vi "LV to text.vi"() -> ()   [LabVIEW 2013]
uses:
  <vilib>/_script/All Supported PropertiesOrMethods TypeDefs/ASC_ArrayOfUniqueIDStringParentIDStringName.ctl
  <vilib>/_script/All Supported PropertiesOrMethods TypeDefs/ASC_UniqueIDStringParentIDStringName.ctl
panel:
  out "Array 5":cluster{i32, "AllTypes[]":T1, "Type":T2}[](array[cluster])
  out "Array 4":cluster{i32, refnum<vi>}[](array[cluster])
  out "const":T3(array[cluster])
  out "Array 2":bool[][](array[boolean])
  out "Array":T4(array[cluster])
  out "nodes":T5(array[cluster])
  out "connectorPane":T6(array[cluster])
  out "NConn":u32
  out "Pattern":u32
  out "SubVIs":T7(array[cluster])
  out "AllObj":T8(array[cluster])
  out "Decorations[]":refnum<vi>[](array[refnum])
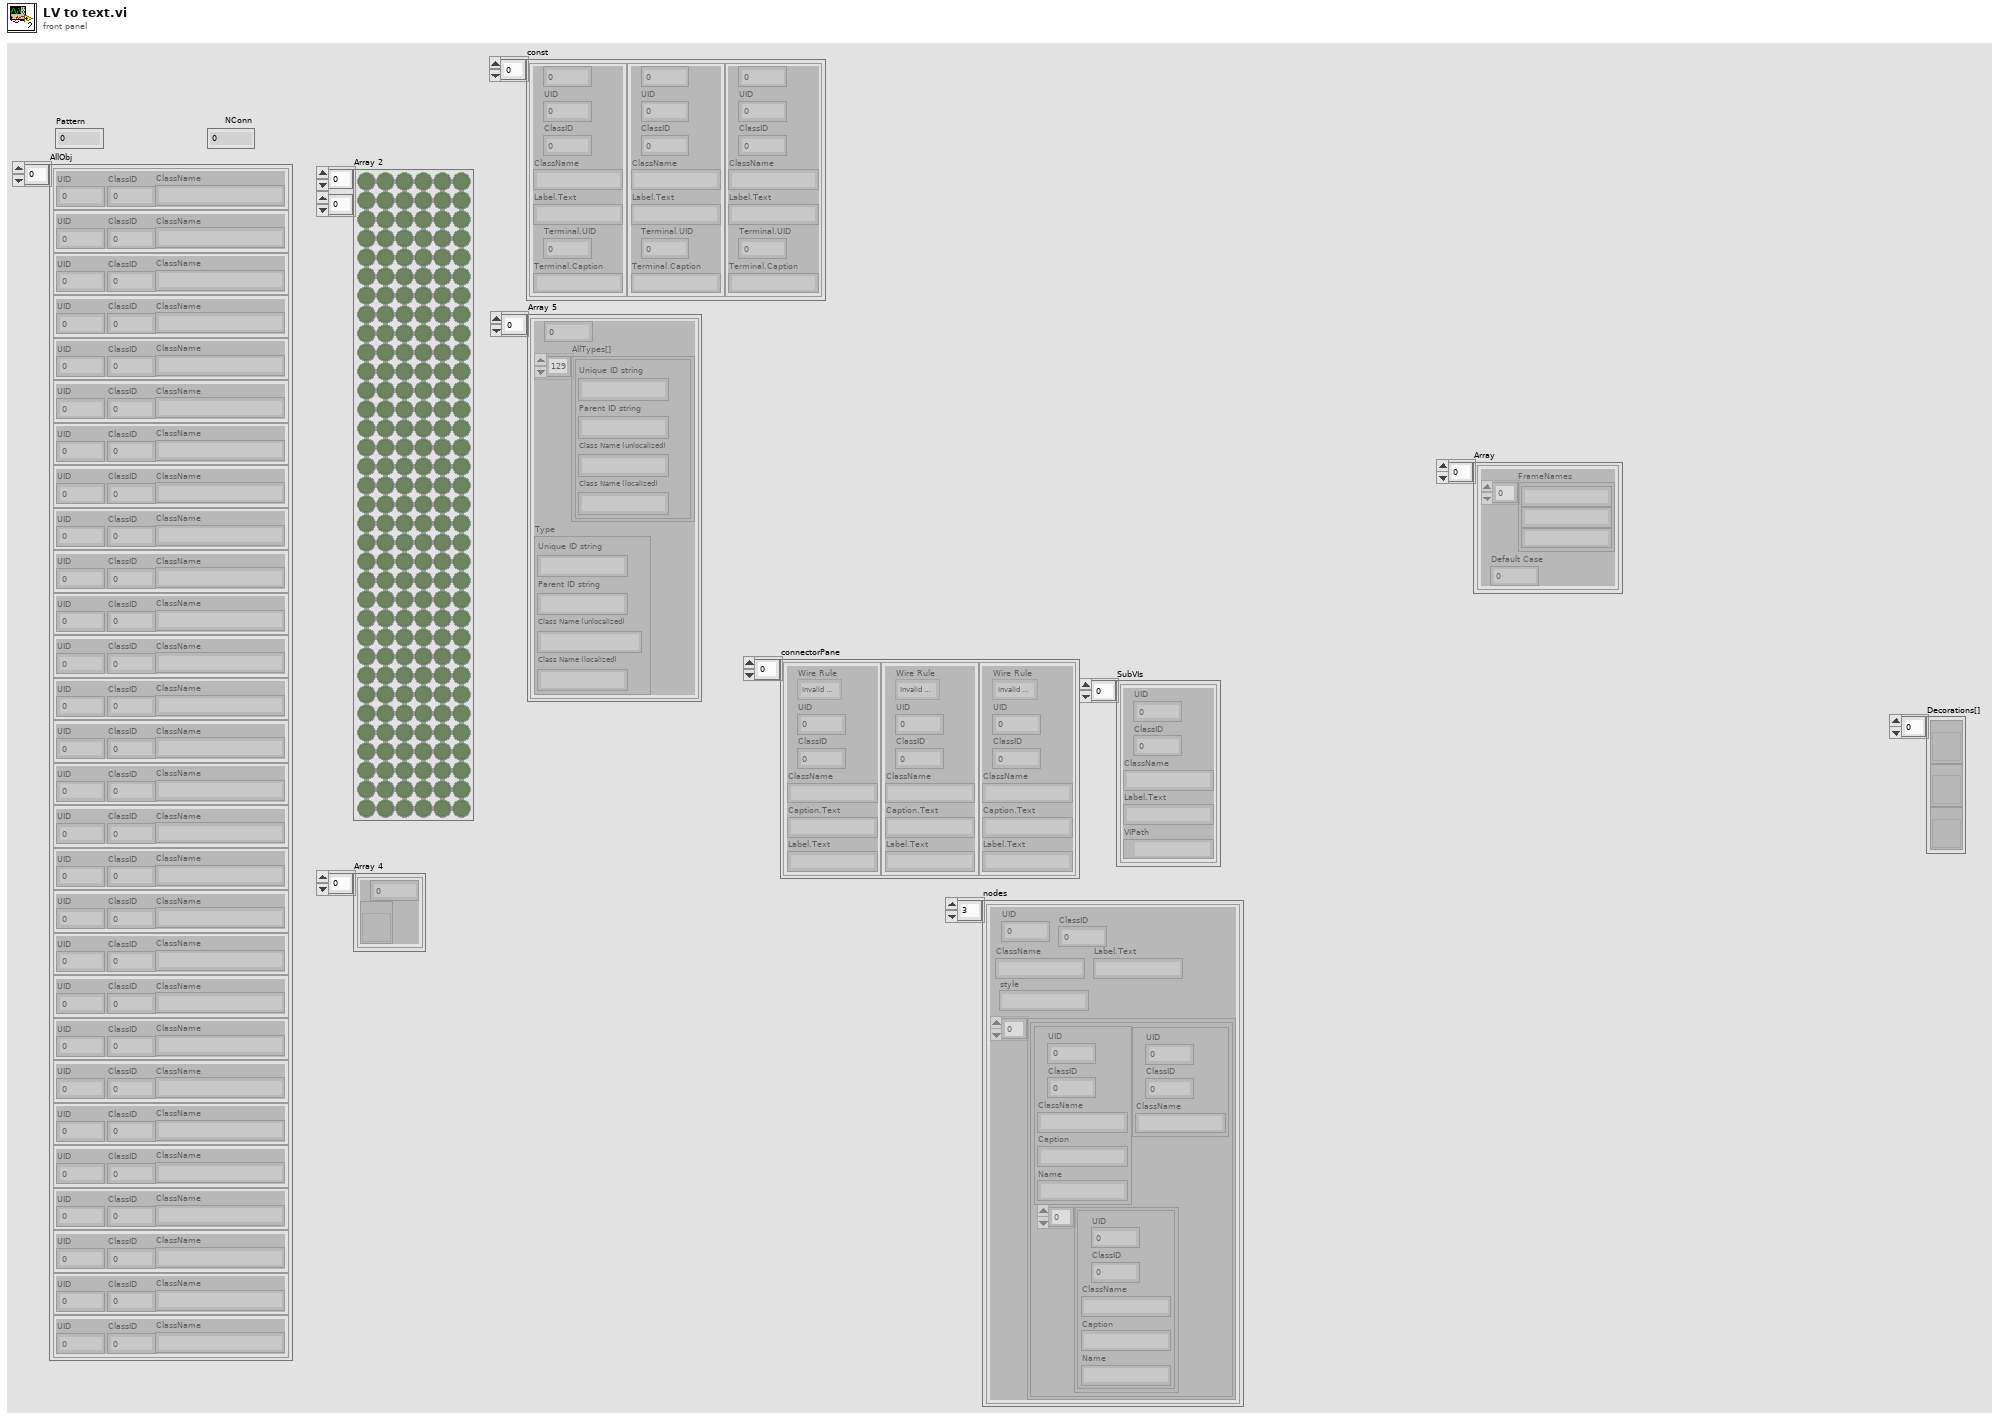
[diagram p1: front panel]
types:
  T1 = typedef "ASC_ArrayOfUniqueIDStringParentIDStringName.ctl" = T2[]
  T2 = typedef "ASC_UniqueIDStringParentIDStringName.ctl" = cluster{"Unique ID string":string, "Parent ID string":string, "Class Name (unlocalized)":string, "Class Name (localized)":string}
  T3 = cluster{i32, "UID":i32, "ClassID":u32, "ClassName":string, "Label.Text":string, "Terminal.UID":i32, "Terminal.Caption":string}[]
  T4 = cluster{"FrameNames":string[], "Default Case":i32}[]
  T5 = cluster{"UID":i32, "ClassID":u32, "ClassName":string, "Label.Text":string, "style":string, cluster{cluster{"UID":i32, "ClassID":u32, "ClassName":string, "Caption":string, "Name":string}, cluster{"UID":i32, "ClassID":u32, "ClassName":string}, cluster{"UID":i32, "ClassID":u32, "ClassName":string, "Caption":string, "Name":string}[]}[]}[]
  T6 = cluster{"Wire Rule":enum16{"Invalid Wire Rule", "Required", "Recommended", "Optional", "Dynamic Dispatch"}, "UID":i32, "ClassID":u32, "ClassName":string, "Caption.Text":string, "Label.Text":string}[]
  T7 = cluster{"UID":i32, "ClassID":u32, "ClassName":string, "Label.Text":string, "VIPath":path}[]
  T8 = cluster{"UID":i32, "ClassID":u32, "ClassName":string}[]
  T9 = enum16{"Invalid Wire Rule", "Required", "Recommended", "Optional", "Dynamic Dispatch"}[]
  T10 = cluster{"Wire Rule":enum16{"Invalid Wire Rule", "Required", "Recommended", "Optional", "Dynamic Dispatch"}, "UID":i32, "ClassID":u32, "ClassName":string, "Caption.Text":string, "Label.Text":string}
  T11 = cluster{"UID":i32, "ClassID":u32, "ClassName":string}
  T12 = cluster{"UID":i32, "ClassID":u32, "ClassName":string, "Caption":string, "Name":string}
  T13 = cluster{cluster{"UID":i32, "ClassID":u32, "ClassName":string, "Caption":string, "Name":string}, cluster{"UID":i32, "ClassID":u32, "ClassName":string}, cluster{"UID":i32, "ClassID":u32, "ClassName":string, "Caption":string, "Name":string}[]}
  T14 = cluster{"UID":i32, "ClassID":u32, "ClassName":string, "Label.Text":string, "Style":string, cluster{cluster{"UID":i32, "ClassID":u32, "ClassName":string, "Caption":string, "Name":string}, cluster{"UID":i32, "ClassID":u32, "ClassName":string}, cluster{"UID":i32, "ClassID":u32, "ClassName":string, "Caption":string, "Name":string}[]}[]}
  T15 = cluster{"UID":i32, "ClassID":u32, "ClassName":string, "Label.Text":string, "VIPath":path}
  T16 = cluster{i32, "UID":i32, "ClassID":u32, "ClassName":string, "Label.Text":string, "Terminal.UID":i32, "Terminal.Caption":string}
  T17 = cluster{"FrameNames":string[], "Default Case":i32}
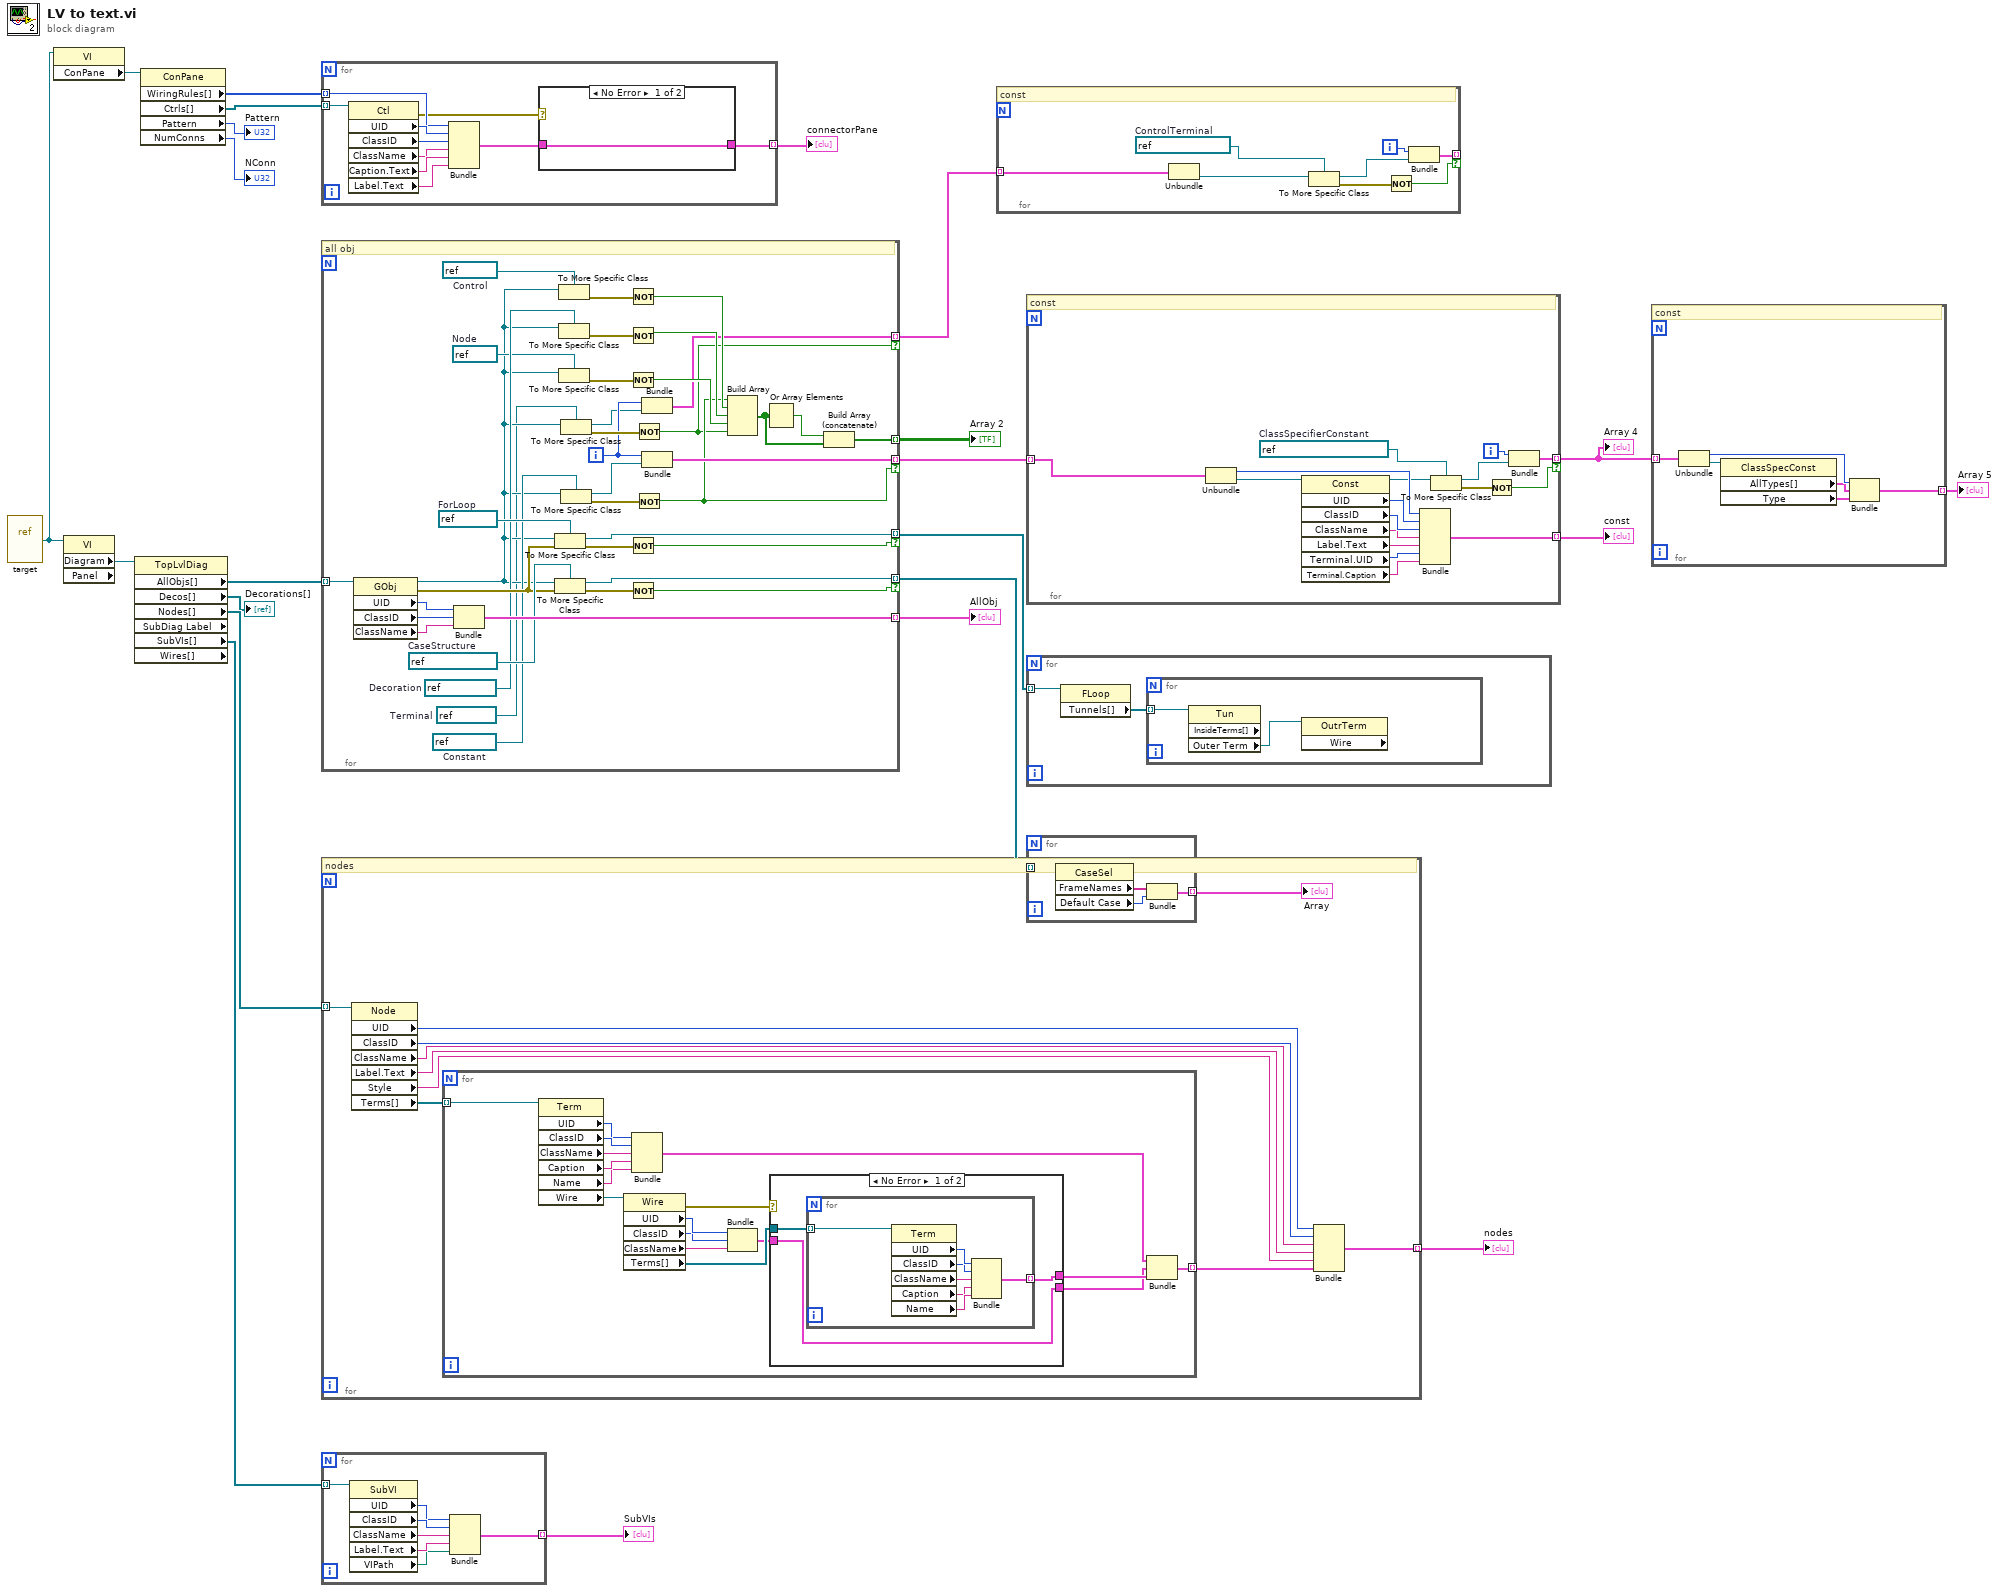
[diagram p0: block diagram]
diagram:
  n1 = vi-ref "target.vi"() -> (w24:refnum<vi>)
  n2 = property class="VI"(reference=w24) -> ("ConPane"=w17:refnum<vi>)  [unwired: 1 in, 2 out]
  n3 = property class="VI" props=["Diagram", "Panel"](reference=w24) -> ("Diagram"=w23:refnum<vi>)  [unwired: 1 in, 3 out]
  n4 = property class="TopLvlDiag" props=["AllObjs[]", "Decos[]", "Nodes[]", "SubDiag Label", "SubVIs[]", "Wires[]"](reference=w23) -> ("AllObjs[]"=w7:refnum<vi>[], "Decos[]"=→"Decorations[]":refnum<vi>[], "Nodes[]"=w22:refnum<vi>[], "SubVIs[]"=w20:refnum<vi>[])  [unwired: 1 in, 4 out]
  n5 = property class="ConPane"(reference=w17) -> ("WiringRules[]"=w14:T9, "Ctrls[]"=w13:refnum<vi>[], "Pattern"=→"Pattern":u32, "NumConns"=→"NConn":u32)  [unwired: 1 in, 2 out]
  n6 = for {
    tunnel: w14 -> [w28] mode=indexing
    tunnel: w13 -> [w29] mode=indexing
    tunnel: [w25] -> w12 mode=indexing
    n7 = property class="Ctl"(reference=w29) -> (error out=w27:errorcluster, "UID"=w30:i32, "ClassID"=w31:u32, "ClassName"=w32:string, "Caption.Text"=w33:string, "Label.Text"=w34:string)  [unwired: 1 in, 1 out]
    n8 = Bundle("Wire Rule"=w28, "UID"=w30, "ClassID"=w31, "ClassName"=w32, "Caption.Text"=w33, "Label.Text"=w34) -> (w26:T10)  [unwired: 1 in]
    n9 = case shown="No Error" w27 {
      tunnel: w26 -> [w35 _]
      tunnel: [w35 _] -> w25
      frame No Error {
      }
      frame Error {
      }
    }
  }
  "connectorPane" <- w12
  n10 = for {
    tunnel: w7 -> [w62] mode=indexing
    tunnel: [w71] -> w19 mode=indexing
    tunnel: [w68] -> w10 mode=indexing if=w52
    tunnel: [w64] -> w8 mode=indexing if=w53
    tunnel: [w41] -> w6 mode=indexing
    tunnel: [w44] -> w5 mode=indexing if=w38
    tunnel: [w39] -> w1 mode=indexing if=w36
    i -> [w40]
    w47 = refnum<vi> refnum  # Terminal
    w58 = refnum<vi> refnum  # Node
    w59 = refnum<vi> refnum  # Decoration
    w60 = refnum<vi> refnum  # Control
    w61 = refnum<vi> refnum  # Constant
    w66 = refnum<vi> refnum  # ForLoop
    w69 = refnum<vi> refnum  # CaseStructure
    # "all obj"
    n11 = property class="GObj"(reference=w62) -> (reference out=w48:refnum<vi>, error out=w65:errorcluster, "UID"=w70:i32, "ClassID"=w73:u32, "ClassName"=w72:string)  [unwired: 1 in]
    n12 = Bundle("UID"=w70, "ClassID"=w73, "ClassName"=w72) -> (w71:T11)  [unwired: 1 in]
    n13 = To More Specific Class(target class=w66, reference=w48, error in=w65) -> (specific class reference=w64:refnum<vi>, error out=w63:errorcluster)
    n14 = To More Specific Class(target class=w69, reference=w48, error in=w65) -> (specific class reference=w68:refnum<vi>, error out=w67:errorcluster)
    n15 = To More Specific Class(target class=w60, reference=w48) -> (error out=w56:errorcluster)  [unwired: 1 in, 1 out]
    n16 = To More Specific Class(target class=w59, reference=w48) -> (error out=w55:errorcluster)  [unwired: 1 in, 1 out]
    n17 = To More Specific Class(target class=w58, reference=w48) -> (error out=w54:errorcluster)  [unwired: 1 in, 1 out]
    n18 = To More Specific Class(target class=w47, reference=w48) -> (specific class reference=w37:refnum<vi>, error out=w46:errorcluster)  [unwired: 1 in]
    n19 = To More Specific Class(target class=w61, reference=w48) -> (specific class reference=w45:refnum<vi>, error out=w57:errorcluster)  [unwired: 1 in]
    n20 = Not(x=w56) -> (.not. x?=w51:bool)
    n21 = Not(x=w55) -> (.not. x?=w50:bool)
    n22 = Not(x=w54) -> (.not. x?=w49:bool)
    n23 = Not(x=w63) -> (.not. x?=w53:bool)
    n24 = Not(x=w67) -> (.not. x?=w52:bool)
    n25 = Not(x=w46) -> (.not. x?=w36:bool)
    n26 = Not(x=w57) -> (.not. x?=w38:bool)
    n27 = Bundle(w40, w37) -> (w39:cluster{i32, refnum<vi>})  [unwired: 1 in]
    n28 = Bundle(w40, w45) -> (w44:cluster{i32, refnum<vi>})  [unwired: 1 in]
    n29 = Build Array(w38, w51, w50, w49, w36) -> (w43:bool[])
    n30 = Or Array Elements(Boolean array=w43) -> (logical OR=w42:bool)
    n31 = Build Array (concatenate)(w42, w43) -> (w41:bool[])
  }
  "AllObj" <- w19
  "Array 2" <- w6
  n32 = for {
    tunnel: w22 -> [w77] mode=indexing
    tunnel: [w80] -> w11 mode=indexing
    # "nodes"
    n33 = property class="Node"(reference=w77) -> ("UID"=w76:i32, "ClassID"=w82:u32, "ClassName"=w81:string, "Label.Text"=w79:string, "Style"=w74:string, "Terms[]"=w78:refnum<vi>[])  [unwired: 1 in, 2 out]
    n34 = for {
      tunnel: w78 -> [w99] mode=indexing
      tunnel: [w87] -> w75 mode=indexing
      n35 = property class="Term"(reference=w99) -> ("UID"=w94:i32, "ClassID"=w98:u32, "ClassName"=w97:string, "Caption"=w96:string, "Name"=w95:string, "Wire"=w93:refnum<vi>)  [unwired: 1 in, 2 out]
      n36 = property class="Wire"(reference=w93) -> (error out=w83:errorcluster, "UID"=w92:i32, "ClassID"=w91:u32, "ClassName"=w90:string, "Terms[]"=w89:refnum<vi>[])  [unwired: 1 in, 1 out]
      n37 = Bundle("UID"=w94, "ClassID"=w98, "ClassName"=w97, "Caption"=w96, "Name"=w95) -> (w88:T12)  [unwired: 1 in]
      n38 = Bundle("UID"=w92, "ClassID"=w91, "ClassName"=w90) -> (w85:T11)  [unwired: 1 in]
      n39 = case shown="No Error" w83 {
        tunnel: w89 -> [w102 _]
        tunnel: [w101 _] -> w86
        tunnel: w85 -> [w100 _]
        tunnel: [w100 _] -> w84
        frame No Error {
          n40 = for {
            tunnel: w102 -> [w104] mode=indexing
            tunnel: [w103] -> w101 mode=indexing
            n41 = property class="Term"(reference=w104) -> ("UID"=w109:i32, "ClassID"=w105:u32, "ClassName"=w106:string, "Caption"=w107:string, "Name"=w108:string)  [unwired: 1 in, 2 out]
            n42 = Bundle("UID"=w109, "ClassID"=w105, "ClassName"=w106, "Caption"=w107, "Name"=w108) -> (w103:T12)  [unwired: 1 in]
          }
        }
        frame Error {
        }
      }
      n43 = Bundle(w88, w84, w86) -> (w87:T13)  [unwired: 1 in]
    }
    n44 = Bundle("UID"=w76, "ClassID"=w82, "ClassName"=w81, "Label.Text"=w79, "Style"=w74, w75) -> (w80:T14)  [unwired: 1 in]
  }
  "nodes" <- w11
  n45 = for {
    tunnel: w20 -> [w116] mode=indexing
    tunnel: [w113] -> w18 mode=indexing
    n46 = property class="SubVI"(reference=w116) -> ("UID"=w110:i32, "ClassID"=w115:u32, "ClassName"=w114:string, "Label.Text"=w112:string, "VIPath"=w111:path)  [unwired: 1 in, 2 out]
    n47 = Bundle("UID"=w110, "ClassID"=w115, "ClassName"=w114, "Label.Text"=w112, "VIPath"=w111) -> (w113:T15)  [unwired: 1 in]
  }
  "SubVIs" <- w18
  n48 = for {
    tunnel: w1 -> [w124] mode=indexing
    tunnel: [w120] -> _ mode=indexing if=w119
    i -> [w121]
    w123 = refnum<vi> refnum  # ControlTerminal
    # "const"
    n49 = Unbundle(w124) -> (w117:refnum<vi>)  [unwired: 1 out]
    n50 = To More Specific Class(target class=w123, reference=w117) -> (specific class reference=w118:refnum<vi>, error out=w122:errorcluster)  [unwired: 1 in]
    n51 = Not(x=w122) -> (.not. x?=w119:bool)
    n52 = Bundle(w121, w118) -> (w120:cluster{i32, refnum<vi>})  [unwired: 1 in]
  }
  n53 = for {
    tunnel: w5 -> [w141] mode=indexing
    tunnel: [w132] -> w4 mode=indexing
    tunnel: [w127] -> w3 mode=indexing if=w126
    i -> [w128]
    w131 = refnum<vi> refnum  # ClassSpecifierConstant
    # "const"
    n54 = Unbundle(w141) -> (w139:i32, w140:refnum<vi>)
    n55 = property class="Const"(reference=w140) -> (reference out=w130:refnum<vi>, "UID"=w138:i32, "ClassID"=w137:u32, "ClassName"=w136:string, "Label.Text"=w135:string, "Terminal.UID"=w134:i32, "Terminal.Caption"=w133:string)  [unwired: 1 in, 1 out]
    n56 = Bundle(w139, "UID"=w138, "ClassID"=w137, "ClassName"=w136, "Label.Text"=w135, "Terminal.UID"=w134, "Terminal.Caption"=w133) -> (w132:T16)  [unwired: 1 in]
    n57 = To More Specific Class(target class=w131, reference=w130) -> (specific class reference=w125:refnum<vi>, error out=w129:errorcluster)  [unwired: 1 in]
    n58 = Not(x=w129) -> (.not. x?=w126:bool)
    n59 = Bundle(w128, w125) -> (w127:cluster{i32, refnum<vi>})  [unwired: 1 in]
  }
  "const" <- w4
  "Array 4" <- w3
  n60 = for {
    tunnel: w8 -> [w143] mode=indexing
    n61 = property class="FLoop"(reference=w143) -> ("Tunnels[]"=w142:refnum<vi>[])  [unwired: 1 in, 2 out]
    n62 = for {
      tunnel: w142 -> [w145] mode=indexing
      n63 = property class="Tun" props=["InsideTerms[]", "Outer Term"](reference=w145) -> ("Outer Term"=w144:refnum<vi>)  [unwired: 1 in, 3 out]
      n64 = property class="OutrTerm" props=["Wire"](reference=w144) -> ()  [unwired: 1 in, 3 out]
    }
  }
  n65 = for {
    tunnel: w10 -> [w149] mode=indexing
    tunnel: [w146] -> w9 mode=indexing
    n66 = property class="CaseSel"(reference=w149) -> ("FrameNames"=w148:string[], "Default Case"=w147:i32)  [unwired: 1 in, 2 out]
    n67 = Bundle("FrameNames"=w148, "Default Case"=w147) -> (w146:T17)  [unwired: 1 in]
  }
  "Array" <- w9
  n68 = for {
    tunnel: w3 -> [w155] mode=indexing
    tunnel: [w151] -> w2 mode=indexing
    # "const"
    n69 = Unbundle(w155) -> (w154:i32, w150:refnum<vi>)
    n70 = property class="ClassSpecConst"(reference=w150) -> ("AllTypes[]"=w153:T1, "Type"=w152:T2)  [unwired: 1 in, 2 out]
    n71 = Bundle(w154, "AllTypes[]"=w153, "Type"=w152) -> (w151:cluster{i32, "AllTypes[]":T1, "Type":T2})  [unwired: 1 in]
  }
  "Array 5" <- w2
